vi "Do.vi"(8 "error in (no error)":errorcluster, 10 "Actor in":refnum<class "Actor.lvclass">, 11 "Receive Joystick Update Msg":refnum<class "Receive Joystick Update Msg.lvclass">) -> (0 "error out":errorcluster, 2 "Actor out":refnum<class "Actor.lvclass">)   [LabVIEW 2014, in "Comp XBox One Controller.lvlib" / "Receive Joystick Update Msg.lvclass"]
doc: "This VI delivers the message to the actor by calling the appropriate method(s) on the actor."
uses:
  Receive Joystick Update Msg.lvclass
  <vilib>/ActorFramework/Actor/Actor.lvclass
  Test-XBox Controller-Receive Updates/Test-XBox Controller-Receive Updates.lvclass
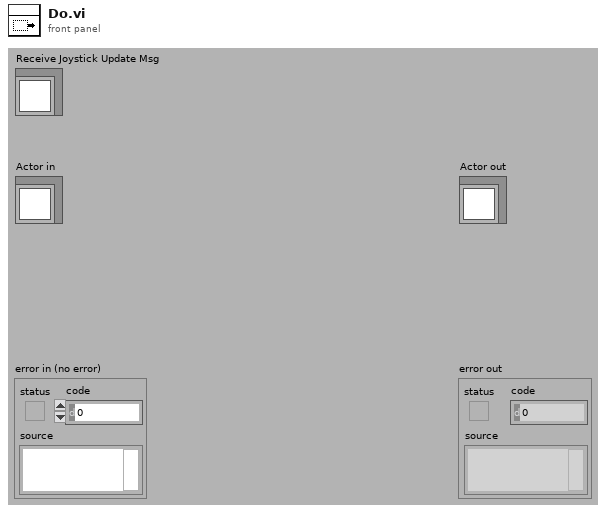
[diagram p1: front panel]
types:
  T1 = typedef "Joystick.lvlib/Joystick.lvclass/Joystick State.ctl" = cluster{"Buttons":T2[], "Axis":T3[]}
  T2 = typedef "Joystick.lvlib/Joystick.lvclass/Button State.ctl" = cluster{"Pressed":bool, "Instance Name":string, "Toggled":bool, "Just Changed":bool}
  T3 = typedef "Joystick.lvlib/Joystick.lvclass/Axis State.ctl" = cluster{"Instance Name":string, "Deadband":dbl, "Value":dbl, "At Home":bool, "Postive Axis Button State":T2, "Negative Axis Button State":T2, "Home Axis Button State":T2}
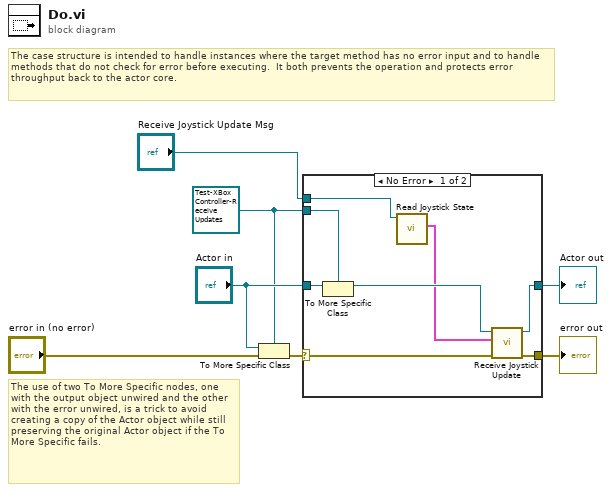
[diagram p0: block diagram]
diagram:
  w2 = refnum<class "Test-XBox Controller-Receive Updates.lvclass"> refnum ("Actor in")
  # "The use of two To More Specific nodes, one with the output object unwired and the other with the error unwired, is a trick to avoid creating a copy of the Actor object while still preserving the original Actor object if the To More Specific fails."
  # "The case structure is intended to handle instances where the target method has no error input and to handle methods that do not check for error before executing.  It both prevents the operation and protects error throughput back to the actor core."
  n1 = To More Specific Class(target class=w2, reference="Actor in", error in="error in (no error)") -> (error out=w6:errorcluster)  [unwired: 1 out]
  n2 = case shown="No Error" w6 {
    selector: w6 -> [w13 w17]
    tunnel: [w15 w17] -> w5
    tunnel: [w14 w16] -> w4
    tunnel: "Actor in" -> [w12 w16]
    tunnel: w2 -> [w11 _]
    tunnel: "Receive Joystick Update Msg" -> [w9 _]
    frame No Error {
      n3 = To More Specific Class(target class=w11, reference=w12) -> (specific class reference=w10:refnum<class "Test-XBox Controller-Receive Updates.lvclass">)  [unwired: 1 in, 1 out]
      n4 = call-dynamic "Read Joystick State.vi"("Get Joystick State Msg in"=w9) -> ("Joystick State"=w8:T1)  [unwired: 8 in, 2 out]
      n5 = call-dynamic "Receive Joystick Update.vi"("error in (no error)"=w13, "Joystick State"=w8, "Test-XBox Controller-Receive Updates in"=w10) -> ("Joystick.lvlib:Joystick.lvclass:Joystick State.ctlerror out"=w15:errorcluster, "Test-XBox Controller-Receive Updates out"=w14:refnum<class "Test-XBox Controller-Receive Updates.lvclass">)  [unwired: 7 in]
    }
    frame Error {
      # "If type check fails, pass the original object out again."
    }
  }
  "error out" <- w5
  "Actor out" <- w4
